vi "Sort ROI data.vi"(8 "ROI numbers":i32[](array[numeric]), 11 "Data for ticked ROI":T1=[{"Plot.Plot Name"="1: Point", "Data"={"X-Axis values"=array[43860 elements], "Y-Axis values (s)"=array[43860 elements]}, "Timeline data"={"X-Axis values"=[], "Y-Axis values (s)"=[]}, "Type"=enum."Mini-scan", "Points per cycle"=1, "ROI number"=0}]) -> (1 "POI raw data":T1, 2 "Miniscan raw data":T1, 3 "Sorted Pointers":i32[](array[numeric]))   [LabVIEW 2013]
uses:
  xcontrol/Interface VIs/Interface typedefs/Interface-Data array.ctl
  xcontrol/Interface VIs/Interface typedefs/Interface-Data format definition.ctl
  xcontrol/Typedefs/Xctl-XY data type definition.ctl
  xcontrol/Typedefs/Xctrl-ROI type enum.ctl
  Program Files (x86)/National Instruments/LabVIEW 2013/user.lib/_OpenG.lib/array/array.llb/Sort 1D Array (I32)__ogtk.vi
  xcontrol/XGrapher.xctl
panel:
  # "<--- This can be used to reorder a concatenated array of any type containing miniscans first followed by POI."
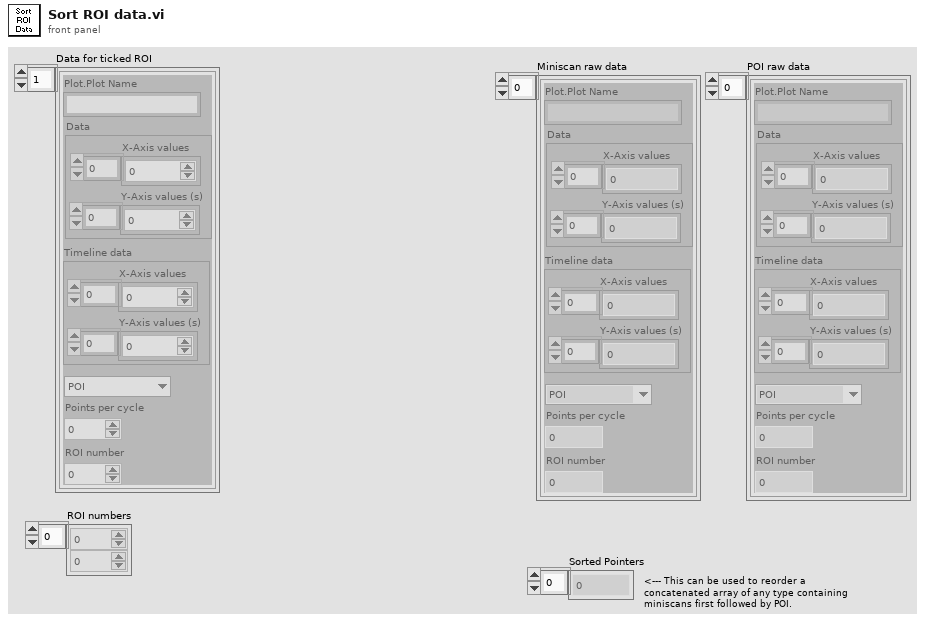
[diagram p1: front panel]
types:
  T1 = typedef "Interface-Data array.ctl" = T2[]
  T2 = typedef "Interface-Data format definition.ctl" = cluster{"Plot.Plot Name":string, "Data":T3, "Timeline data":T3, "Type":T4, "Points per cycle":u16, "ROI number":u16}
  T3 = typedef "XGrapher.xctl/Xctl-XY data type definition.ctl" = cluster{"X-Axis values":sgl[], "Y-Axis values (s)":i32[]}
  T4 = typedef "Xctrl-ROI type enum.ctl" = enum16{"POI", "Mini-scan", "Group"}
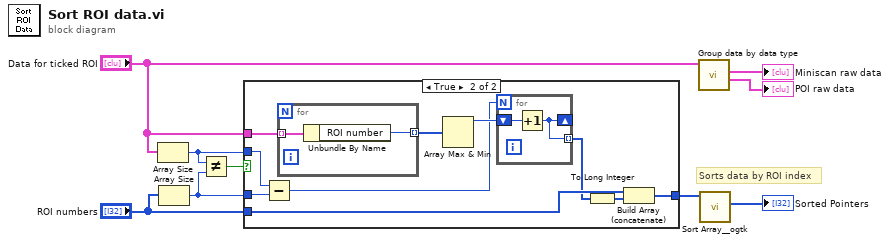
[diagram p0: block diagram]
diagram:
  # "Sorts data by ROI index"
  n1 = Array Size(array="Data for ticked ROI") -> (size(s)=w5:i32)
  n2 = Array Size(array="ROI numbers") -> (size(s)=w1:i32)
  n3 = Not Equal?(x=w5, y=w1) -> (x != y?=w6:bool)
  n4 = case shown="True" w6 {
    tunnel: w5 -> [_ w17]
    tunnel: "ROI numbers" -> [w10 w14]
    tunnel: [w10 w12] -> w3
    tunnel: "Data for ticked ROI" -> [_ w20]
    tunnel: w1 -> [_ w16]
    frame False {
    }
    frame True {
      n5 = Subtract(x=w17, y=w16) -> (x-y=w15:i32)
      n6 = for {
        tunnel: w20 -> [w24] mode=indexing
        tunnel: [w23] -> w19 mode=indexing
        n7 = Unbundle By Name(w24) -> ("ROI number"=w23:u16)
      }
      n8 = Array Max & Min(array=w19) -> (max value=w18:u16)  [unwired: 3 out]
      n9 = for {
        N: w15 -> [_]
        shift-right: [w21] -> _
        shift-left: w18 -> [w22]
        tunnel: [w21] -> w13 mode=indexing
        n10 = Increment(x=w22) -> (x+1=w21:u16)
      }
      n11 = To Long Integer(number=w13) -> (32bit integer=w11:i32[])
      n12 = Build Array (concatenate)(w14, w11) -> (w12:i32[])
    }
  }
  n13 = call "Group data by data type.vi"("Raw data"="Data for ticked ROI") -> ("POI data"=→"POI raw data":T1, "Miniscan data"=→"Miniscan raw data":T1)  [unwired: 8 in, 1 out]
  n14 = call-poly "Sort Array__ogtk.vi"("Array in"=w3) -> ("Sorted Pointers"=→"Sorted Pointers":i32[])  [unwired: 9 in, 1 out]
